vi "Read Temperature (DegF).vi"(8 "error in (no error)":errorcluster, 11 "HTS221 in":refnum<class "HTS221.lvclass">) -> (0 "error out":errorcluster, 2 "Temperature (degF)":dbl, 3 "HTS221 out":refnum<class "HTS221.lvclass">)   [LabVIEW 2020, in "HTS221.lvclass"]
uses:
  HTS221.lvclass
  HTS221.lvclass/HTS221.ctl
  Read Temperature.Zero.vi
  Read Temperature.Slope.vi
  LINX I2C/LINX I2C.lvclass
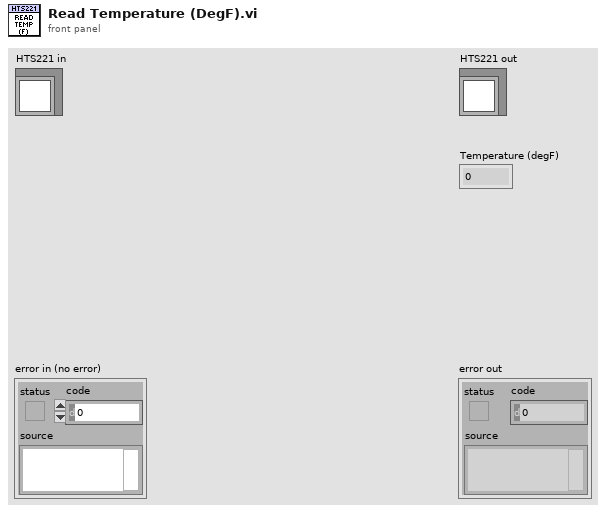
[diagram p1: front panel]
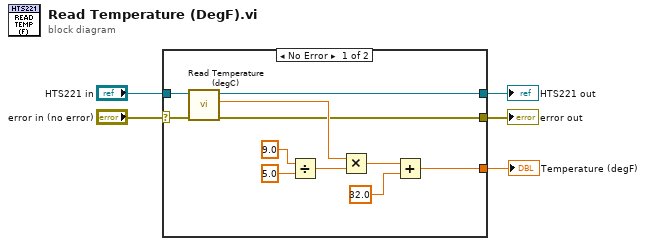
[diagram p0: block diagram]
diagram:
  n1 = case shown="No Error" "error in (no error)" {
    selector: "error in (no error)" -> [w16 w18]
    tunnel: [w7 w18] -> w4
    tunnel: [w6 w17] -> w2
    tunnel: "HTS221 in" -> [w15 w17]
    tunnel: [w8 _] -> w1
    frame No Error {
      n2 = call "Read Temperature (degC).vi"("error in (no error)"=w16, "HTS221 in"=w15) -> ("error out"=w7:errorcluster, "Temperature (degC)"=w14:dbl, "HTS221 out"=w6:refnum<class "HTS221.lvclass">)  [unwired: 7 in]
      n3 = Divide(x=9.0 ("y"), y=5.0) -> (x/y=w11:dbl)
      n4 = Multiply(x=w14, y=w11) -> (x*y=w10:dbl)
      n5 = Add(x=w10, y=32.0) -> (x+y=w8:dbl)
    }
    frame Error {
    }
  }
  "error out" <- w4
  "HTS221 out" <- w2
  "Temperature (degF)" <- w1
